vi "sub_vi_calibration.vi"(8 "error in (no error)":errorcluster, 10 "Gain":u16, 11 "VISA resource name":refnum<visa-resource-name>) -> (0 "error out":errorcluster, 1 "Weights":dbl[](array[numeric]), 2 "Measures":dbl[](array[numeric]), 3 "VISA resource name out":refnum<visa-resource-name>, 4 "Relative errors array":dbl[](array[numeric]), 5 "Calibration - read data":dbl[][](array[numeric]), 6 "Absolute errors array":dbl[](array[numeric]), 7 "Noise":dbl[](array[numeric]))   [LabVIEW 2016]
uses:
  <vilib>/Analysis/NI_AALBase.lvlib
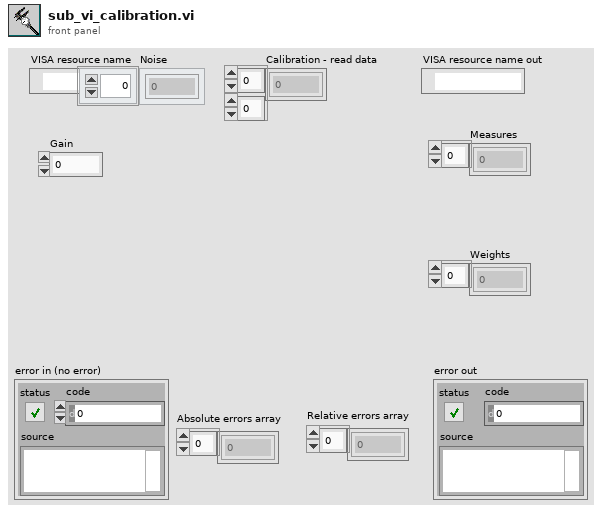
[diagram p1: front panel]
types:
  T1 = cluster{"[0]":dbl, "[1]":dbl, "[2]":dbl, "[3]":dbl, "[4]":dbl, "[5]":dbl, "[6]":dbl, "[7]":dbl, "[8]":dbl}
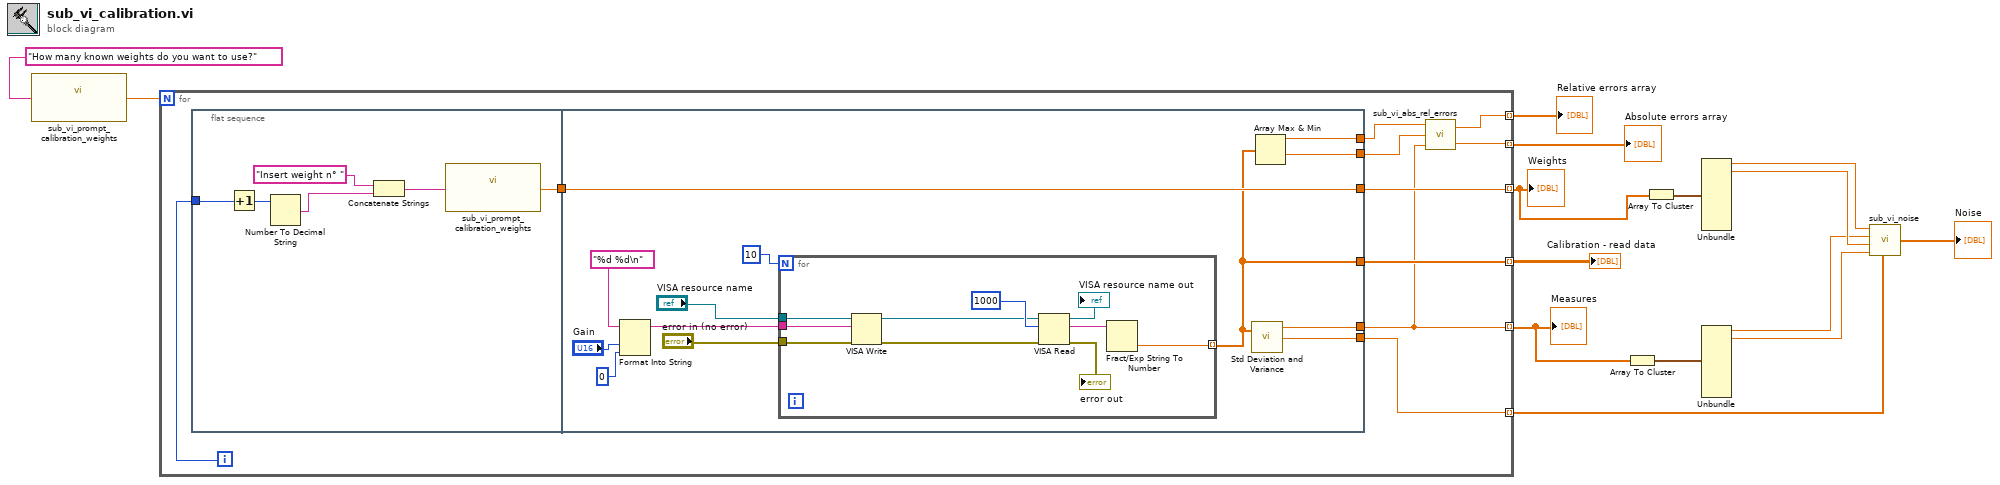
[diagram p0: block diagram]
diagram:
  n1 = call "sub_vi_prompt_calibration_weights.vi"("Title"="How many known weights do you want to use?") -> ("Weights number 2"=w14:dbl)  [unwired: 18 in]
  n2 = for {
    N: w14 -> [_]
    tunnel: [w22] -> w10 mode=indexing
    tunnel: [w19] -> w3 mode=indexing
    tunnel: [w23] -> w13 mode=indexing
    tunnel: [w20] -> w12 mode=indexing
    tunnel: [w21] -> w11 mode=indexing
    tunnel: [w16] -> w1 mode=indexing
    i -> [w25]
    n3 = flat-sequence {
      tunnel: w25 -> [w28]
      tunnel: [w26] -> w24
      tunnel: [w44] -> w22
      tunnel: w24 -> [w44]
      tunnel: [w33] -> w19
      tunnel: [w34] -> w23
      tunnel: [w36] -> w18
      tunnel: [w35] -> w17
      tunnel: [w32] -> w16
      frame #0 {
        n4 = Increment(x=w28) -> (x+1=w31:i32)
        n5 = Number To Decimal String(number=w31) -> (decimal integer string=w30:string)  [unwired: 1 in]
        n6 = Concatenate Strings("Insert weight n° ", w30) -> (w29:string)
        n7 = call "sub_vi_prompt_calibration_weights.vi"("Title"=w29) -> ("Weights number 2"=w26:dbl)  [unwired: 18 in]
      }
      frame #1 {
        n8 = Format Into String(format string="%d %d\n", "Gain", u16 0 ("input 2")) -> (resulting string=w38:string)  [unwired: 2 in, 1 out]
        n9 = for {
          N: 10 -> [_]
          tunnel: [w50] -> w34 mode=indexing
          tunnel: "error in (no error)" -> [w49]
          tunnel: w38 -> [w48]
          tunnel: "VISA resource name" -> [w47]
          n10 = VISA Write(VISA resource name=w47, write buffer=w48, error in (no error)=w49) -> (VISA resource name out=w45:refnum<visa-resource-name>, error out=w46:errorcluster)  [unwired: 1 out]
          n11 = VISA Read(VISA resource name=w45, byte count=u32 1000, error in (no error)=w46) -> (VISA resource name out=→"VISA resource name out":refnum<visa-resource-name>, read buffer=w53:string, error out=→"error out":errorcluster)  [unwired: 1 out]
          n12 = Fract/Exp String To Number(string=w53) -> (number=w50:dbl)  [unwired: 3 in, 1 out]
        }
        n13 = call <vilib>:"Std Deviation and Variance.vi"("X"=w34) -> ("mean"=w33:dbl, "standard deviation"=w32:dbl)  [unwired: 1 in, 1 out]
        n14 = Array Max & Min(array=w34) -> (max value=w36:dbl, min value=w35:dbl)  [unwired: 2 out]
      }
    }
    n15 = call "sub_vi_abs_rel_errors.vi"("Measure"=w19, "Min"=w17, "Max"=w18) -> ("Relative error"=w20:dbl, "Absolute error"=w21:dbl)
  }
  "Weights" <- w10
  "Measures" <- w3
  "Calibration - read data" <- w13
  "Absolute errors array" <- w12
  "Relative errors array" <- w11
  n16 = Array To Cluster(array=w3) -> (cluster=w6:T1)
  n17 = Array To Cluster(array=w10) -> (cluster=w9:T1)
  n18 = Unbundle(w9) -> ("[0]"=w8:dbl, "[1]"=w7:dbl)  [unwired: 7 out]
  n19 = Unbundle(w6) -> ("[0]"=w5:dbl, "[1]"=w4:dbl)  [unwired: 7 out]
  n20 = call "sub_vi_noise.vi"("x1"=w8, "y1"=w5, "x2"=w7, "sigma"=w1, "y2"=w4) -> ("Noise"=→"Noise":dbl[])  [unwired: 3 in]
